vi "ep_Check Data Valid.vi"(0 "waveforms":waveform(dbl)[](array[waveform]), 2 "reset? (F)":bool, 9 "demodulation settings":cluster{"enable? (F)":bool, "algorithm":T1}, 11 "error in (no error)":errorcluster) -> (3 "number of spectra":i32, 4 "signals":dbl[][](array[numeric]), 6 "parameters":T2, 15 "error out":errorcluster)   [LabVIEW 2014, in "NI_EP_Motor Monitoring.lvlib"]
uses:
  <vilib>/addons/Electrical Power/Motor Monitoring/NI_EP_Motor Monitoring.lvlib
  <vilib>/addons/Electrical Power/Motor Monitoring/subVIs/ep_Demodulation Algorithm.ctl
  <vilib>/addons/Electrical Power/Power Measurement/NI_EP_Power Measurement.lvlib
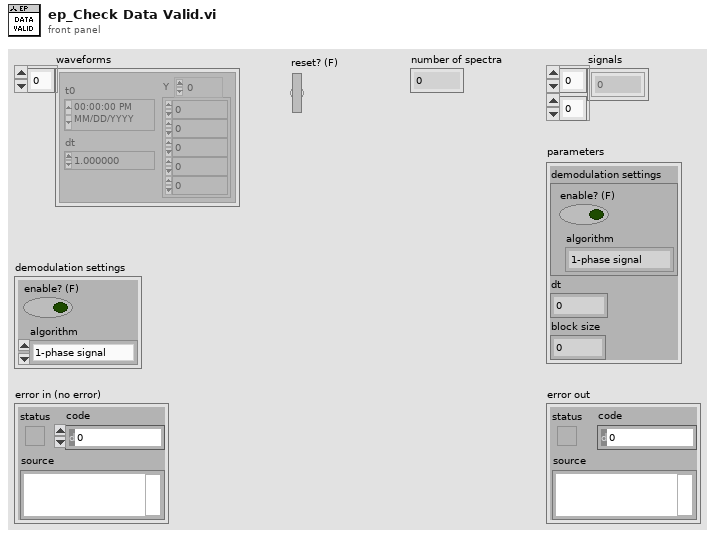
[diagram p1: front panel]
types:
  T1 = typedef "NI_EP_Motor Monitoring.lvlib/ep_Demodulation Algorithm.ctl" = enum16{"1-phase signal", "3-phase signals"}
  T2 = cluster{"demodulation settings":cluster{"enable? (F)":bool, "algorithm":T1}, "dt":dbl, "block size":i32}
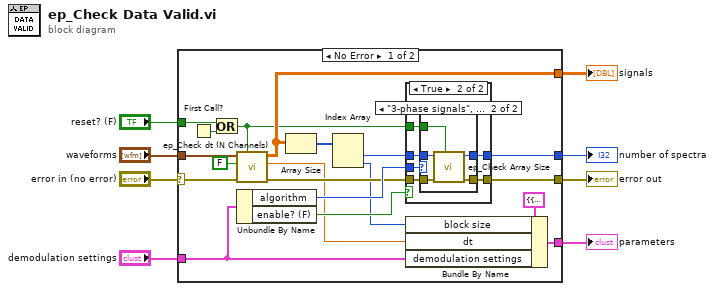
[diagram p0: block diagram]
diagram:
  n1 = case shown="No Error" "error in (no error)" {
    selector: "error in (no error)" -> [w21 w43]
    tunnel: [w18 w43] -> w7
    tunnel: "waveforms" -> [w20 _]
    tunnel: "reset? (F)" -> [w19 _]
    tunnel: "demodulation settings" -> [w10 _]
    tunnel: [w17 _] -> w4
    tunnel: [w16 _] -> w3
    tunnel: [w9 _] -> w1
    frame No Error {
      n2 = First Call?() -> (First Call?: T/F=w23:bool)
      n3 = Or(x=w19, y=w23) -> (x .or. y?=w15:bool)
      n4 = call <vilib>:"ep_Check dt (N Channels).vi"("reset? (F)"=w15, "error in (no error)"=w21, "waveforms only? (F)"=FALSE, "waveforms"=w20) -> ("error out"=w14:errorcluster, "dt"=w12:dbl, "signals"=w16:dbl[][])  [unwired: 3 in, 2 out]
      n5 = Unbundle By Name(w10) -> ("algorithm"=w26:T1, "enable? (F)"=w27:bool)
      n6 = Array Size(array=w16) -> (size(s)=w24:i32[])
      n7 = Index Array(array=w24) -> (element #1=w25:i32, element #2=w11:i32)  [unwired: 2 in]
      n8 = case shown="True" w27 {
        tunnel: w25 -> [w29 w35]
        tunnel: [w28 w34] -> w18
        tunnel: [w29 w33] -> w17
        tunnel: w26 -> [_ w32]
        tunnel: w15 -> [_ w31]
        tunnel: w14 -> [w28 w30]
        frame False {
        }
        frame True {
          n9 = case shown="\"3-phase signals\", Default" w32 {
            tunnel: w35 -> [w37 w42]
            tunnel: [w36 w41] -> w34
            tunnel: [w37 w40] -> w33
            tunnel: w31 -> [_ w39]
            tunnel: w30 -> [w36 w38]
            frame "1-phase signal" {
            }
            frame "3-phase signals", Default {
              n10 = call <vilib>:"ep_Check Array Size.vi"("reset? (F)"=w39, "error in (no error)"=w38, "number of channels"=w42) -> ("error out"=w41:errorcluster, "number of 3 phases"=w40:i32)  [unwired: 7 in]
            }
          }
        }
      }
      n11 = Bundle By Name(cluster=T2 {"demodulation settings"={"enable? (F)"=FALSE, "algorithm"=enum."1-phase signal"}, "dt"=0.0, "block size"=0} ("parameters"), "block size"=w11, "dt"=w12, "demodulation settings"=w10) -> (w9:T2)
    }
    frame Error {
    }
  }
  "error out" <- w7
  "number of spectra" <- w4
  "signals" <- w3
  "parameters" <- w1
